vi "Teleop.vi"() -> ()   [LabVIEW 2012]
doc: "This VI is called for each TeleOp packet received from the DS where the robot is not disabled. It is often used to read from the joysticks and update I/O or to update setpoints for timed control loops. It should complete and return within 20 milliseconds or it may miss DS packets."
uses:
  <vilib>/Rock Robotics/SystemInterfaces/Typedef/FPGA_TypedefAnalogModuleForGyro.ctl
  <vilib>/Rock Robotics/SystemInterfaces/AI/FPGA_AIGyroChannel.ctl
  <vilib>/Rock Robotics/SystemInterfaces/Typedef/FPGA_TypedefDigitalModule.ctl
  Program Files (x86)/National Instruments/LabVIEW 2012/examples/FRC/I2C/ADXL345 I2C/Driver/ADXL345 I2C Range.ctl
  Program Files (x86)/National Instruments/LabVIEW 2012/examples/FRC/I2C/ADXL345 I2C/Driver/ADXL345 I2C Axis.ctl
panel:
  out "Y Displacememt":dbl
  out "Y Velocity":dbl
  out "XDisplacememt":dbl
  out "X Velocity":dbl
  out "Y Acceleration":dbl
  out "X Acceleration":dbl
  out "Angular Rate":dbl
  out "Angle":dbl
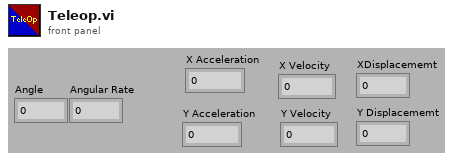
[diagram p1: front panel]
types:
  T1 = typedef "ADXL345 I2C Range.ctl" = u8
  T2 = typedef "FPGA_TypedefDigitalModule.ctl" = enum16{"Digital Module 1", "Digital Module 2"}
  T3 = typedef "FPGA_AIGyroChannel.ctl" = enum8{"AI 1", "AI 2", "Invalid"}
  T4 = typedef "FPGA_TypedefAnalogModuleForGyro.ctl" = enum16{"Analog Module 1"}
  T5 = typedef "WPI_GyroDevRef.ctl" = cluster{"DevStatus":errorcluster, "Analog Module":T6, "Analog Channel":T7, "Offset":dbl, "Gain (VoltsPerDegree/Second)":dbl}
  T6 = typedef "FPGA_TypedefAnalogModule.ctl" = enum16{"Analog Module 1", "Analog Module 2"}
  T7 = typedef "FPGA_AIChannel.ctl" = enum8{"AI 1", "AI 2", "AI 3", "AI 4", "AI 5", "AI 6", "AI 7", "AI 8", "Invalid"}
  T8 = typedef "WPI_I2CDevRef.ctl" = cluster{"DevStatus":errorcluster, "Digital Module":T2, "Device Address":u8}
  T9 = typedef "ADXL345 I2C Axis.ctl" = u8
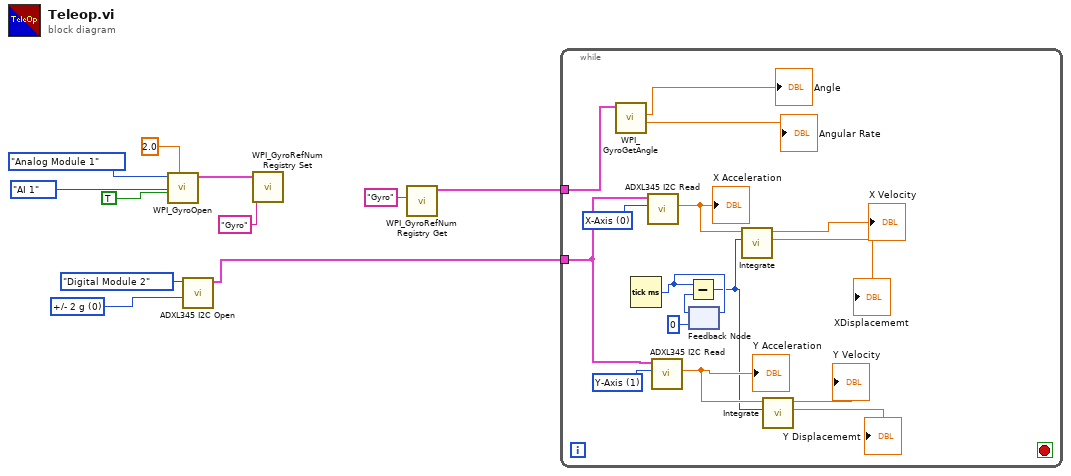
[diagram p0: block diagram]
diagram:
  w2 = T1 0 items=["+/- 2 g", "+/- 4 g", "+/- 8 g", "+/- 16 g"] ("Range")
  n1 = call <vilib>:"WPI_GyroOpen.vi"("Calibration Time (s)"=2.0, "Calibrate On Open"=TRUE, "Analog Channel"=FPGA_AIGyroChannel."AI 1", "Analog Module (Module 1)"=FPGA_TypedefAnalogModuleForGyro."Analog Module 1") -> ("GyroDevRef"=w7:T5)  [unwired: 5 in, 2 out]
  n2 = call "ADXL345 I2C Open.vi"("Range"=w2, "DIO Module (Module 1)"=FPGA_TypedefDigitalModule."Digital Module 2") -> ("I2CDevRef"=w1:T8)  [unwired: 8 in, 1 out]
  n3 = call <vilib>:"WPI_GyroRefNum Registry Set.vi"("refnum name"="Gyro", "GyroDevRef"=w7) -> ()  [unwired: 8 in, 2 out]
  n4 = call <vilib>:"WPI_GyroRefNum Registry Get.vi"("refnum name"="Gyro") -> ("GyroDevRef"=w4:T5)  [unwired: 9 in, 1 out]
  n5 = while {
    tunnel: w4 -> [w27]
    tunnel: w1 -> [w24]
    stop <- _ stop-if-true
    w22 = T9 1 items=["X-Axis", "Y-Axis", "Z-Axis"] ("Axis")
    w23 = T9 0 items=["X-Axis", "Y-Axis", "Z-Axis"] ("Axis")
    n6 = call <vilib>:"WPI_GyroGetAngle.vi"("GyroDevRef"=w27) -> ("Angular Rate"=→"Angular Rate":dbl, "Angle"=→"Angle":dbl)  [unwired: 7 in, 2 out]
    n7 = Tick Count (ms)() -> (millisecond timer value=w19:u32)
    n8 = call "ADXL345 I2C Read.vi"("Axis"=w23, "I2CDevRef"=w24) -> ("Acceleration"=w20:dbl)  [unwired: 7 in, 2 out]
    "X Acceleration" <- w20
    n9 = call "ADXL345 I2C Read.vi"("Axis"=w22, "I2CDevRef"=w24) -> ("Acceleration"=w21:dbl)  [unwired: 7 in, 2 out]
    "Y Acceleration" <- w21
    n10 = feedback-in #1(w19) -> ()
    n11 = feedback #1(u32 0 ("millisecond timer value")) -> (w18:u32)
    n12 = Subtract(x=w19, y=w18) -> (x-y=w16:u32)
    n13 = call "Integrate.vi"("dt"=w16, "Acceleration"=w20) -> ("Displacememt"=→"XDisplacememt":dbl, "Velocity"=→"X Velocity":dbl)  [unwired: 8 in]
    n14 = call "Integrate.vi"("dt"=w16, "Acceleration"=w21) -> ("Displacememt"=→"Y Displacememt":dbl, "Velocity"=→"Y Velocity":dbl)  [unwired: 8 in]
  }
